vi "send_laser_command.vi"(8 "error in (no error)":errorcluster, 11 "String":string="test") -> (0 "error out":errorcluster, 3 "data out":string)   [LabVIEW 2023]
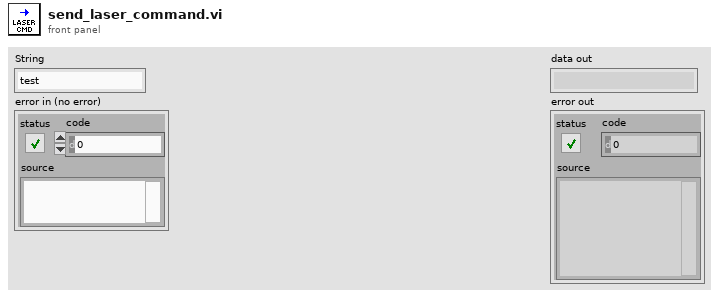
[diagram p1: front panel]
types:
  T1 = enum16{"Standard", "Buffered", "CRLF", "Immediate"}
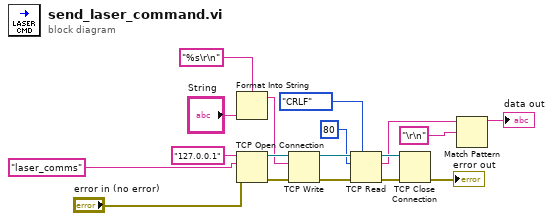
[diagram p0: block diagram]
diagram:
  n1 = Format Into String(format string="%s\r\n", "String") -> (resulting string=w9:string)  [unwired: 2 in, 1 out]
  n2 = TCP Open Connection(address="127.0.0.1", remote port or service name="laser_comms", error in (no error)="error in (no error)") -> (connection ID=w18:refnum<k5>, error out=w17:errorcluster)  [unwired: 2 in]
  n3 = TCP Write(connection ID=w18, data in=w9, error in (no error)=w17) -> (connection ID out=w16:refnum<k5>, error out=w15:errorcluster)  [unwired: 1 in, 1 out]
  n4 = TCP Read(connection ID=w16, bytes to read=80, error in (no error)=w15, 7:T1."CRLF" ("mode (standard)")) -> (connection ID out=w8:refnum<k5>, data out=w3:string, error out=w7:errorcluster)  [unwired: 1 in]
  n5 = TCP Close Connection(connection ID=w8, error in (no error)=w7) -> (error out=→"error out":errorcluster)  [unwired: 1 in, 1 out]
  n6 = Match Pattern(string=w3, regular expression="\r\n" ("format string")) -> (before substring=→"data out":string)  [unwired: 1 in, 3 out]
